vi "数据查询筛选弹框.vi"(8 "error in (no error)":errorcluster caption="错误输入（无错误）", 9 "是否初始化":enum16{"init", "keep"}(ring), 10 "database":string="database1.mdb", 11 "table":string(combo)="CODMn") -> (0 "error out":errorcluster caption="错误输出", 1 "确定输出":bool, 2 "显示项":string[](array[string]), 3 "condition":string)   [LabVIEW 2016]
uses:
  <vilib>/addons/database/Auxilliary.llb/DB Tools DataTypes.ctl
  <vilib>/picture/picture.llb/imagedata.ctl
  <vilib>/Utility/miscctls.llb/LVPointTypeDef.ctl
  <vilib>/Utility/sysdir.llb/System Directory Type.ctl
  <vilib>/addons/database/Connection.llb/DB Tools Open Connec (String).vi
  <vilib>/addons/database/Connection.llb/Conn Execute.vi
  <vilib>/addons/database/Recordset.llb/Rec Fetch Recordset Data (R).vi
  <vilib>/addons/database/Recordset.llb/Rec Destroy - Connection.vi
  <userlib>/_OpenG.lib/array/array.llb/Remove Duplicates from 1D Array (String)__ogtk.vi
  <vilib>/addons/database/_DB Variant To Data/Database Variant To Data.xnode
  <vilib>/addons/database/NI_Database_API.lvlib
panel:
  in  "背景图像":T1
  in  "实时分钟小时数据":enum32{"实时数据", "分钟数据", "小时数据"}(radio)
  in  "确定":bool
  out "自定义2single":cluster{"起始范围":string, "截止范围":string}
  out "自定义1single":cluster{"起始范围":string, "截止范围":string}
  out "自定义2筛选条件":string[](array[string])
  out "自定义1筛选条件":string[](array[string])
  in  "标签 2":string="从：\n\n\n至："
  in  "自定义数值结束 2":dbl
  in  "自定义数值起始 2":dbl
  in  "自定义结束时间 2":timestamp(xcontrol)
  in  "自定义起始时间 2":timestamp(xcontrol)
  in  "自定义 2":T2 caption="自定义"
  in  "下拉列表":string(xcontrol)
  in  "标签":string="从：\n\n\n至："
  in  "自定义数值结束":dbl
  in  "自定义数值起始":dbl
  in  "自定义结束时间":timestamp(xcontrol)
  in  "自定义起始时间":timestamp(xcontrol)
  in  "自定义":T2
  in  "下拉列表 2":string(xcontrol)
  out "type":T3[](array[typedef])
  out "所有测量模式":string[](array[string])
  out "数组":string[](array[string])
  out "columns":string[](array[string])
  in  "测量模式":T4
  in  "退出":bool
  in  "清空":bool
  in  "时间标识输入1":timestamp(xcontrol)
  in  "时间标识输入2":timestamp(xcontrol)
  # "时间"
  # "从："
  # "至："
  # "测试模式"
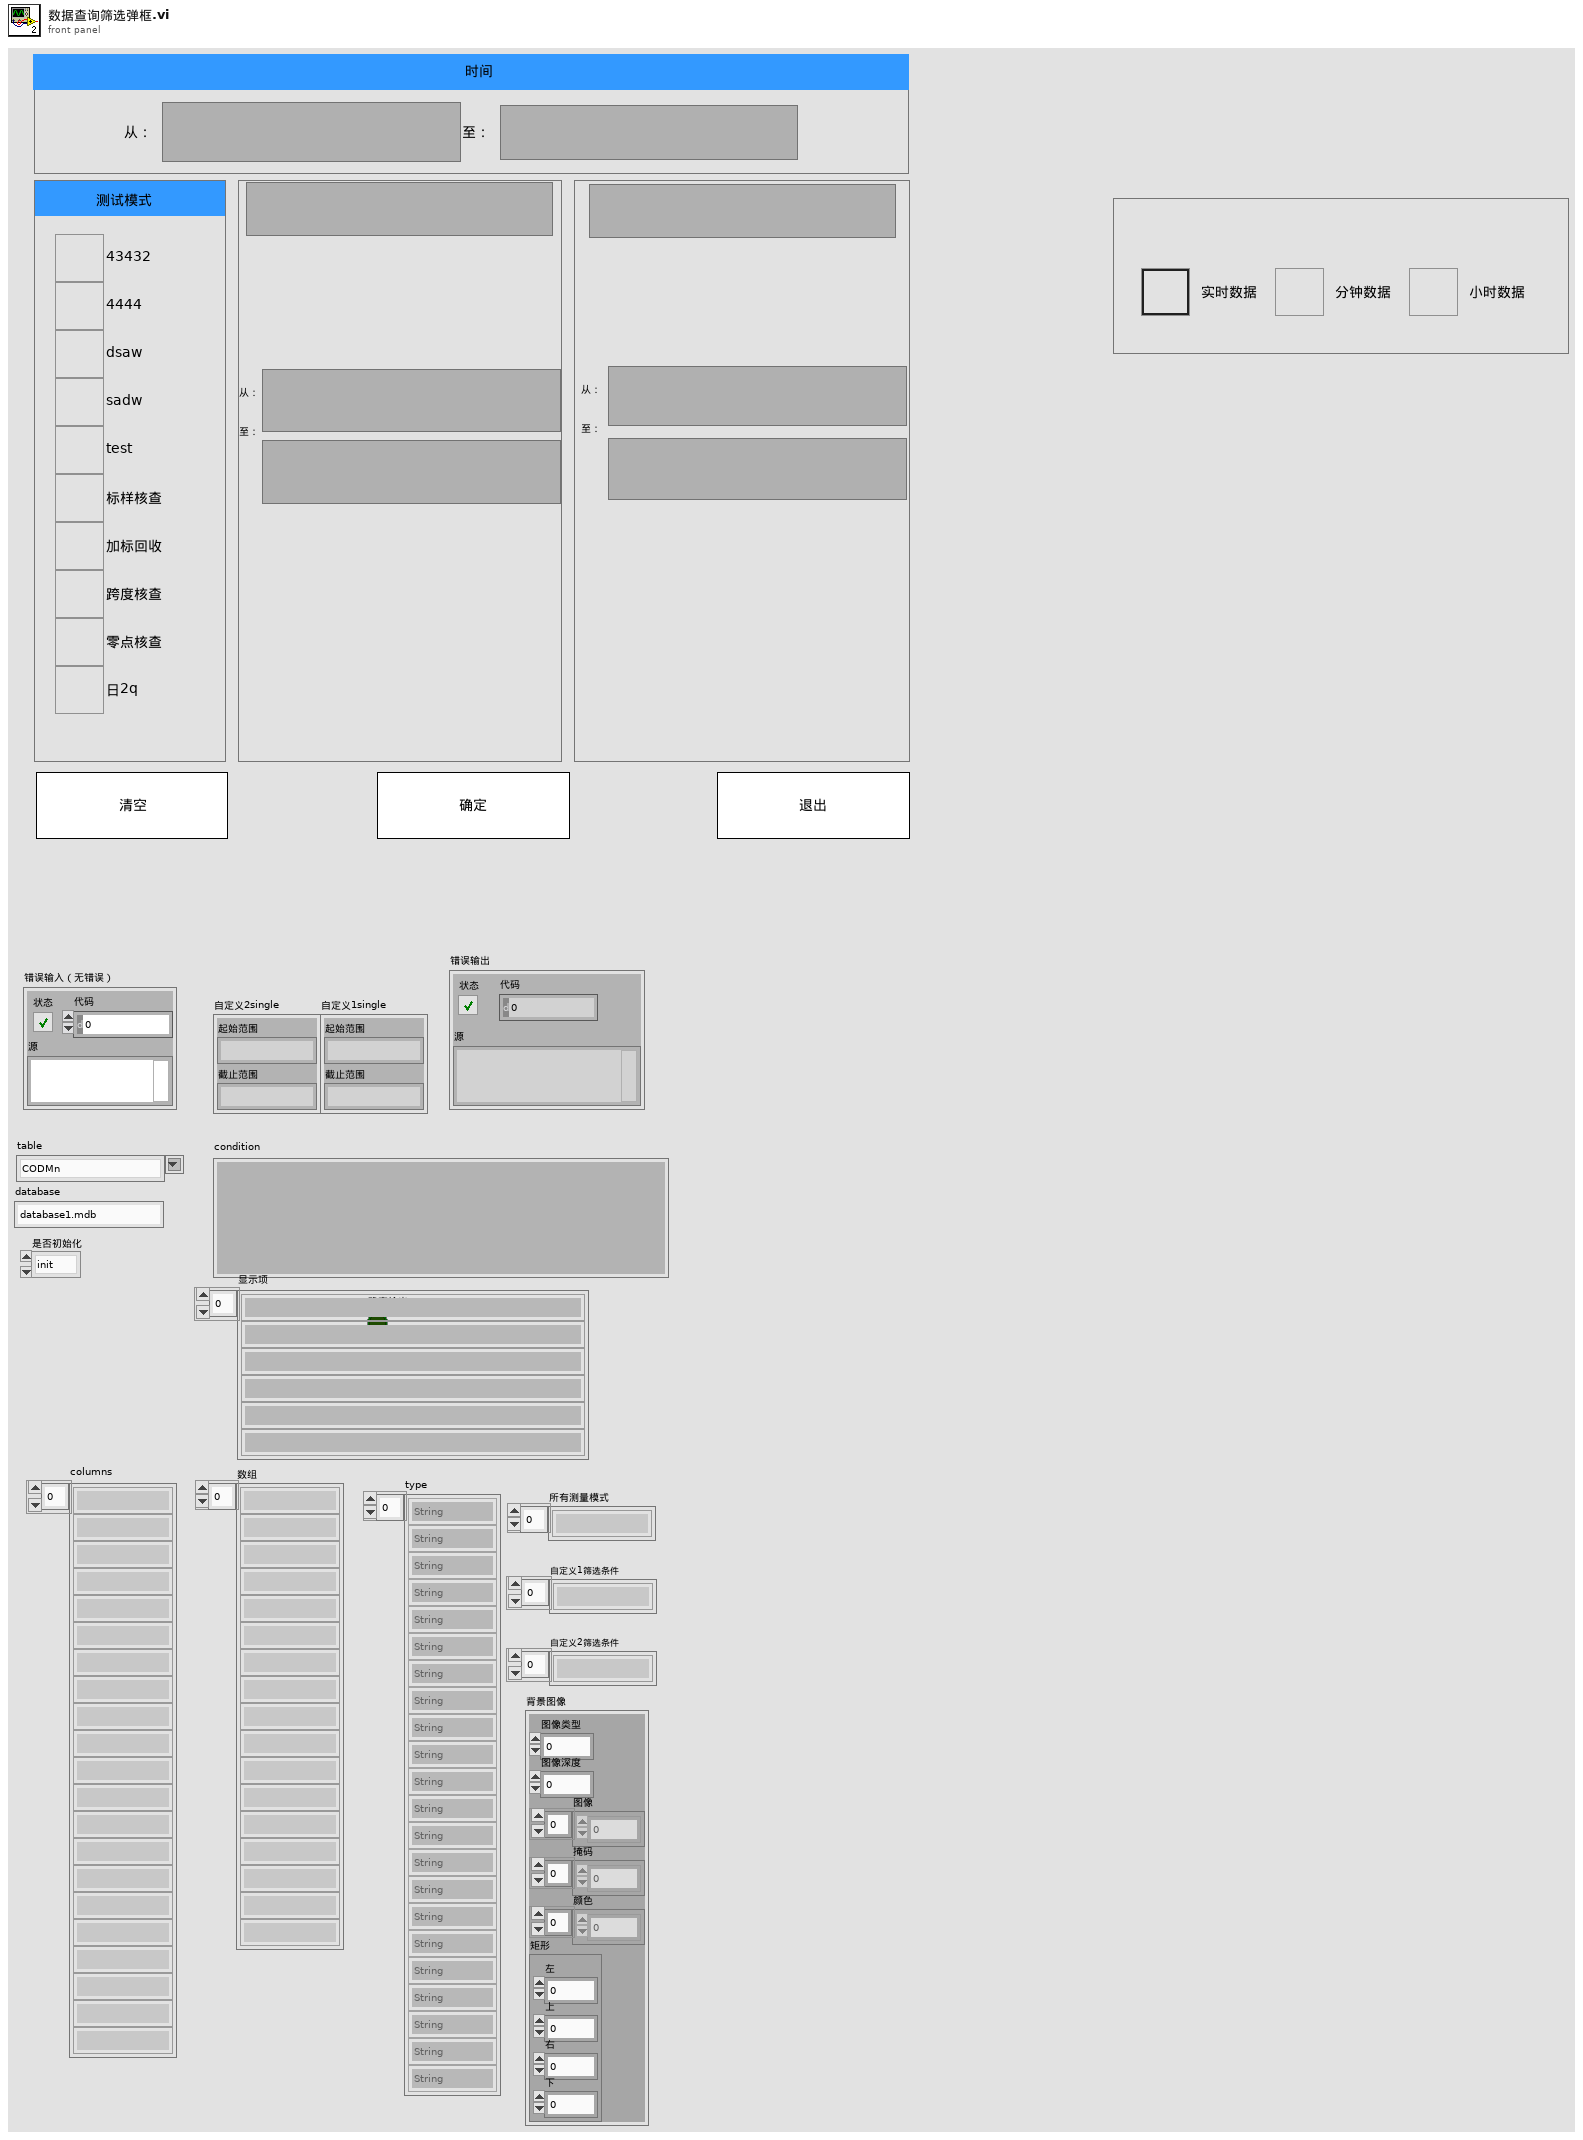
[diagram p1: front panel]
types:
  T1 = typedef "imagedata.ctl" = cluster{"image type":i32, "image depth":i32, "image":u8[], "mask":u8[], "colors":u32[], "Rectangle":cluster{"left":i16, "top":i16, "right":i16, "bottom":i16}}
  T2 = cluster{"DSADSA ":bool, "2":bool, "3":bool, "4":bool, "5":bool, "6":bool, "7":bool, "8":bool, "9":bool, "10":bool}
  T3 = typedef "NI_Database_API.lvlib/DB Tools DataTypes.ctl" = enum16{"String", "Long (I32)", "Single (SGL)", "Double (DBL)", "Date/Time", "Binary"}
  T4 = cluster{"水样测试":bool, "标样核查":bool, "零点核查":bool, "跨度核查":bool, "空白测试":bool, "平行样测试":bool, "加标回收":bool, "空白校准":bool, "标样校准":bool, "初始化清洗":bool}
  T5 = typedef "System Directory Type.ctl" = i32
  T6 = enum8{"Enabled", "Disabled", "Disabled and Grayed Out"}
  T7 = typedef "LVPointTypeDef.ctl" = cluster{"Horizontal":i16, "Vertical":i16}
  T8 = typedef "NI_Database_API.lvlib/Conn ObjectReference.ctl" = refnum<k1>
  T9 = cluster{"name":string, "database data type":T3, "defined size":i32}[]
  T10 = typedef "NI_Database_API.lvlib/Rec ObjectReference.ctl" = refnum<k1>
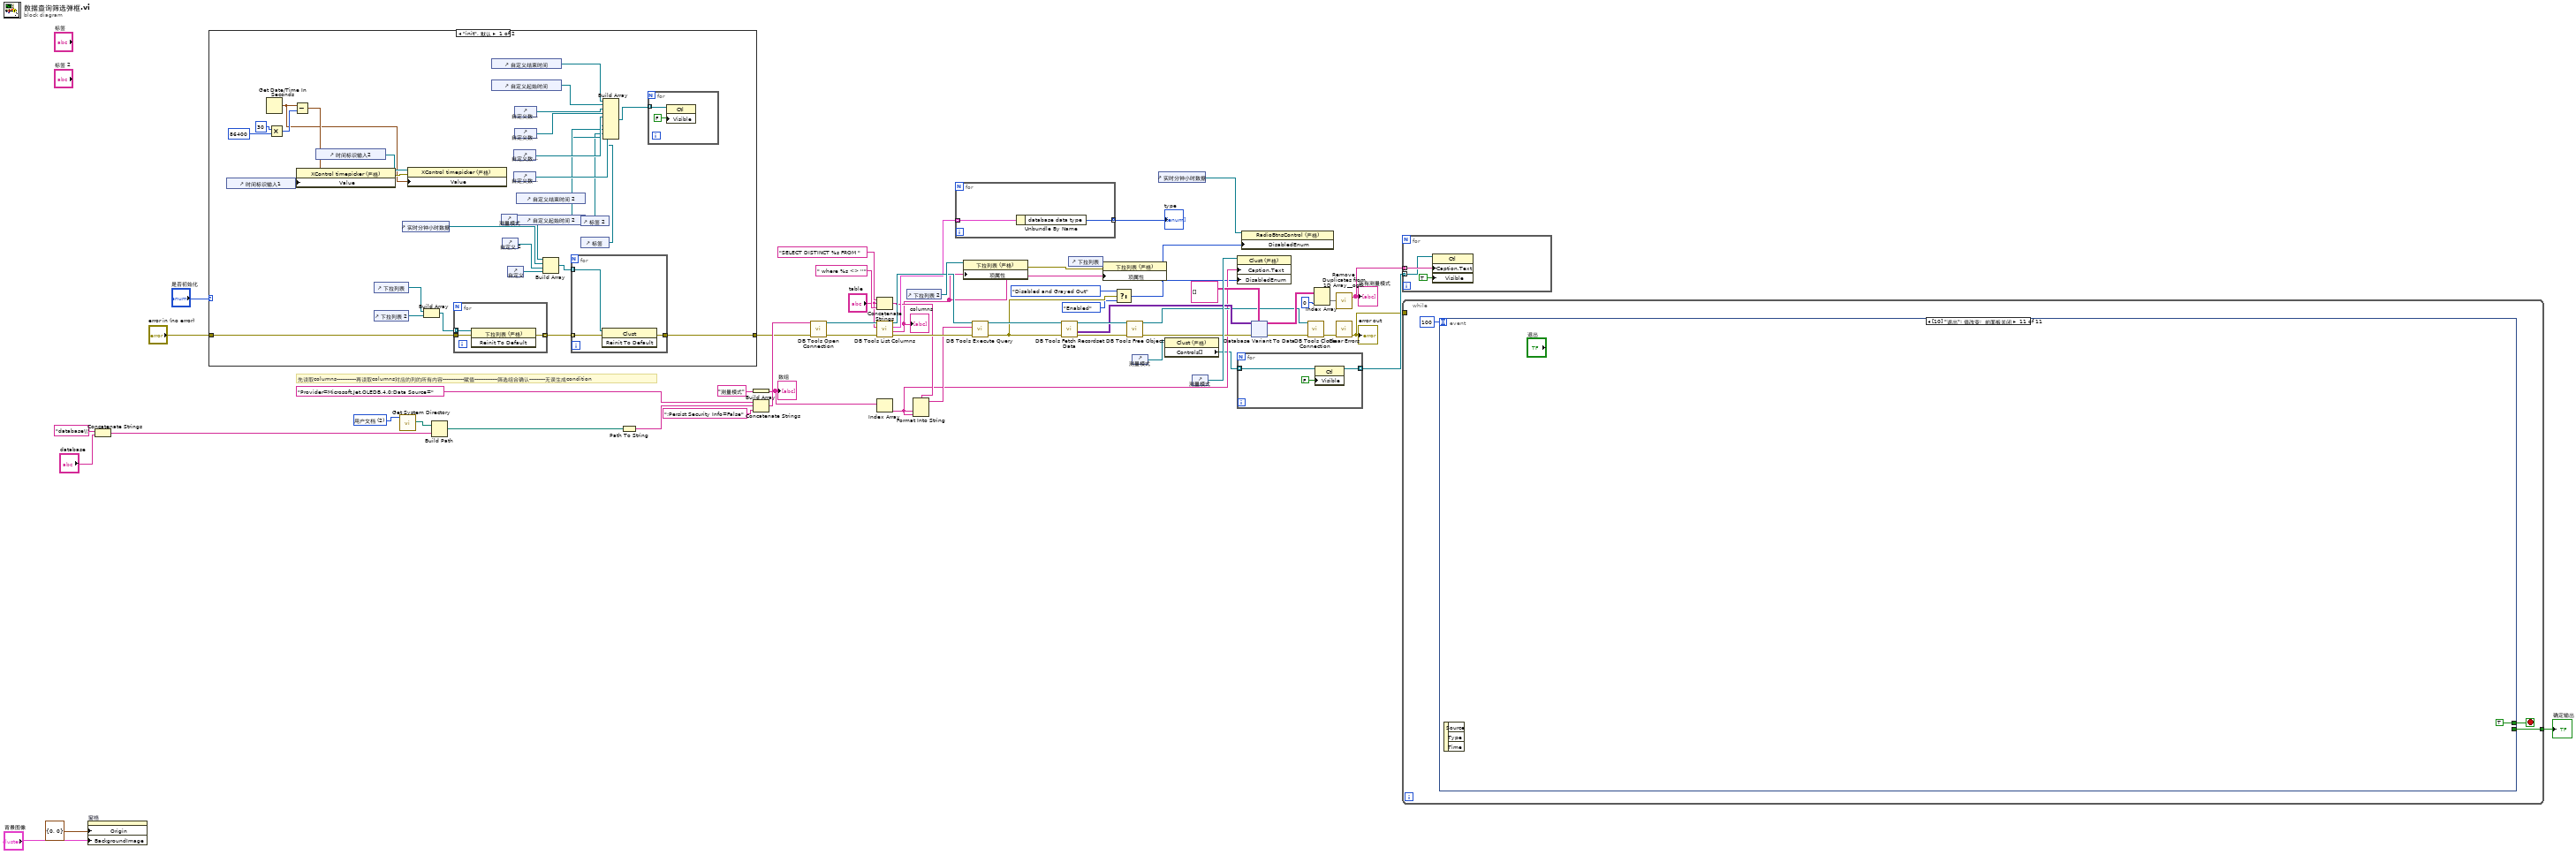
[diagram p0: block diagram]
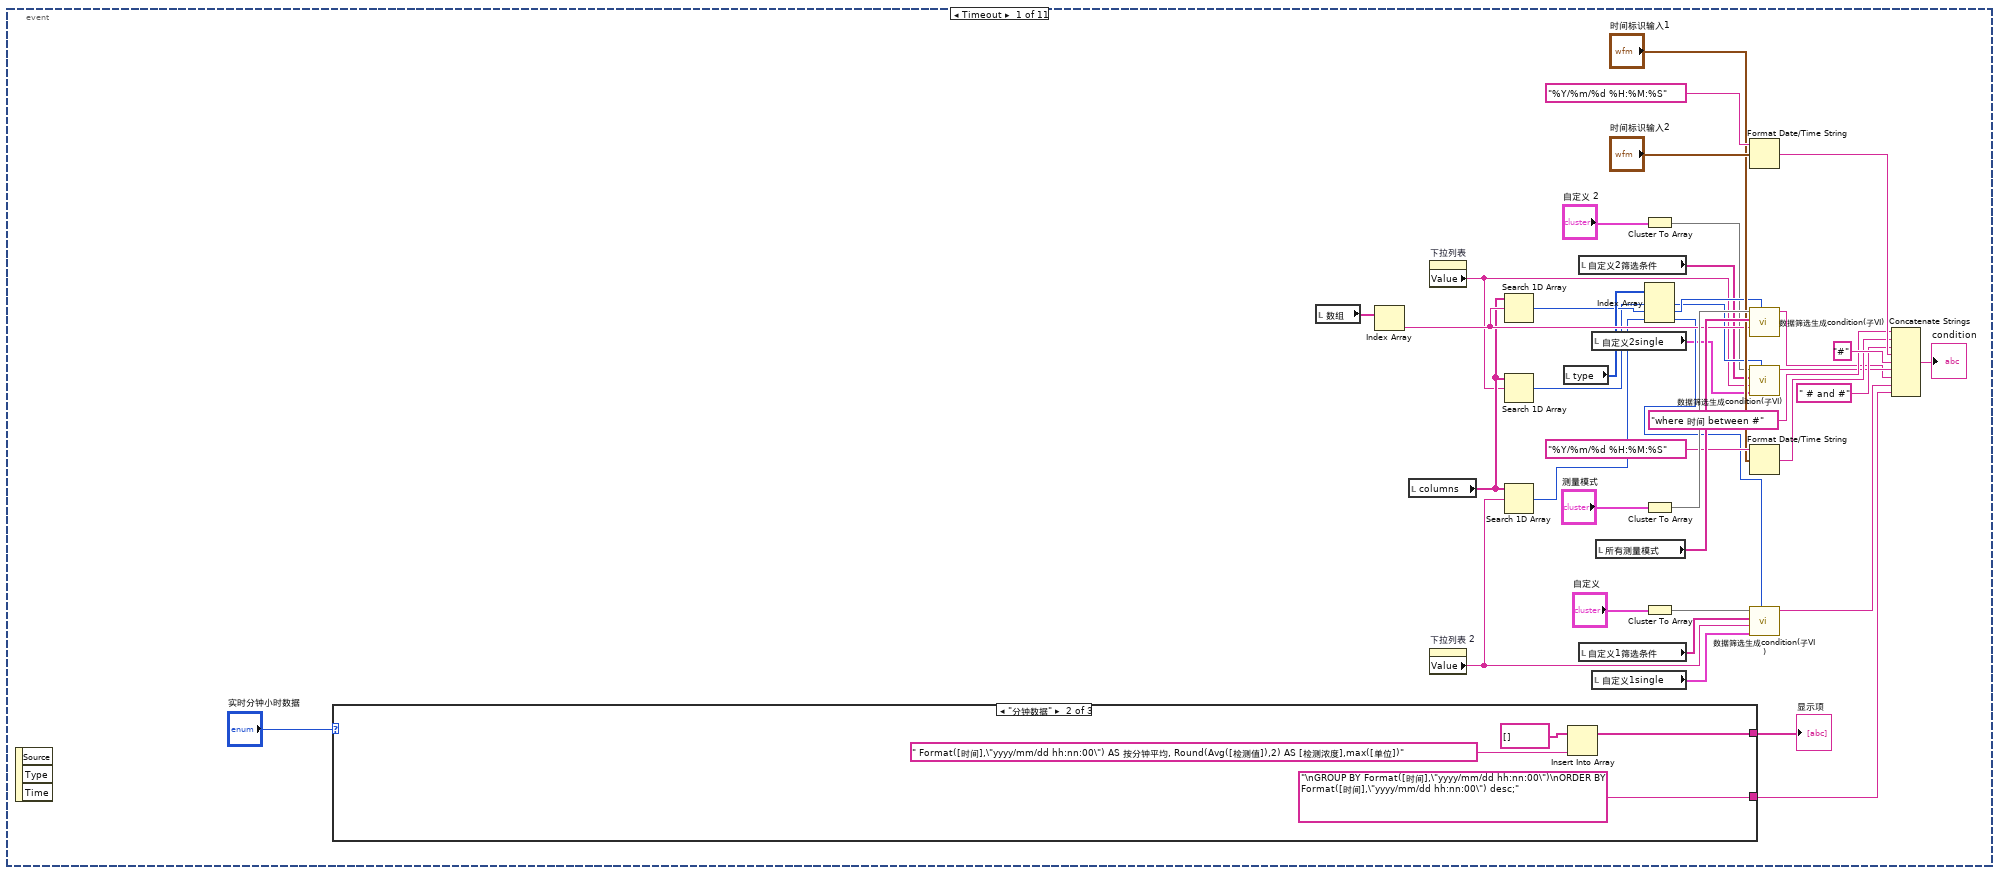
[diagram p3: hidden frame]
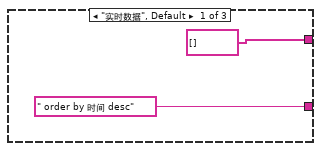
[diagram p4: hidden frame]
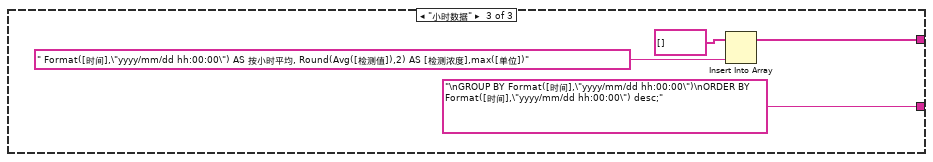
[diagram p5: hidden frame]
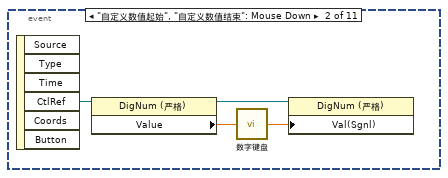
[diagram p6: hidden frame]
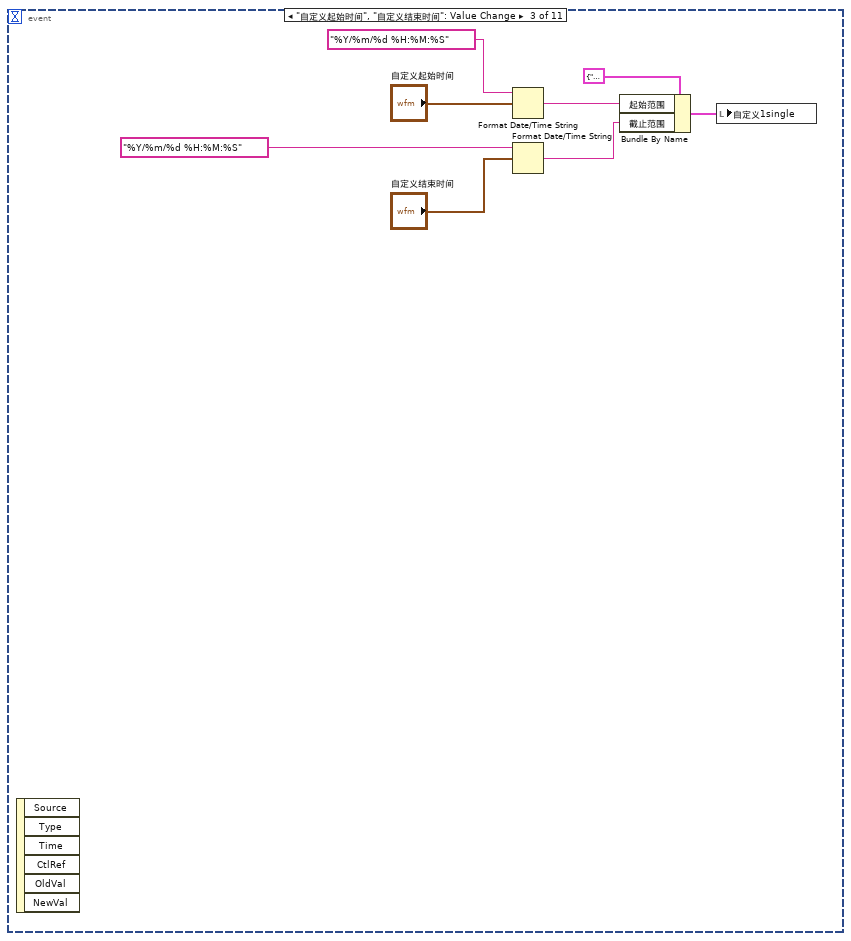
[diagram p7: hidden frame]
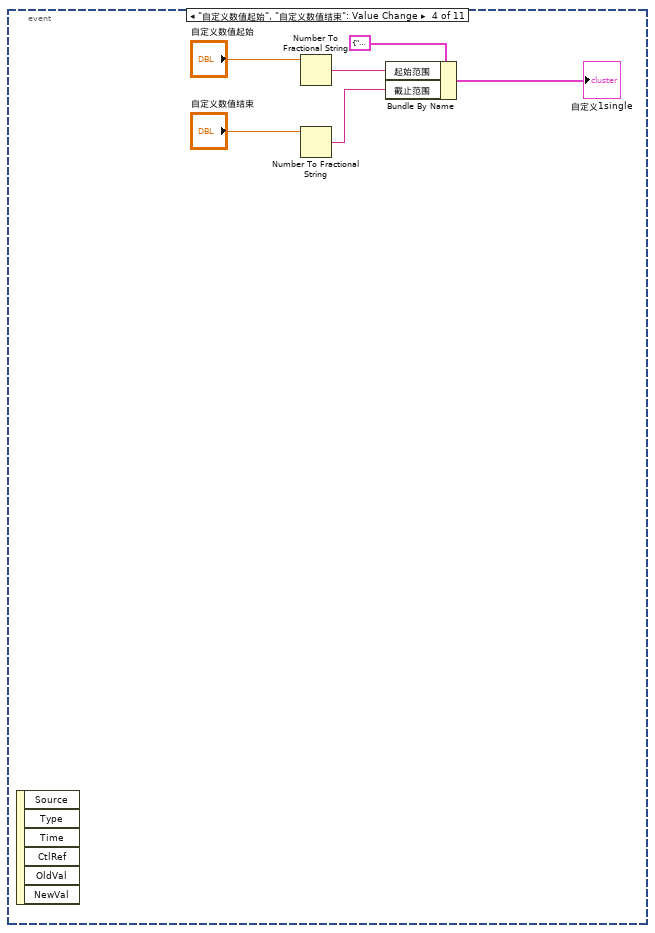
[diagram p8: hidden frame]
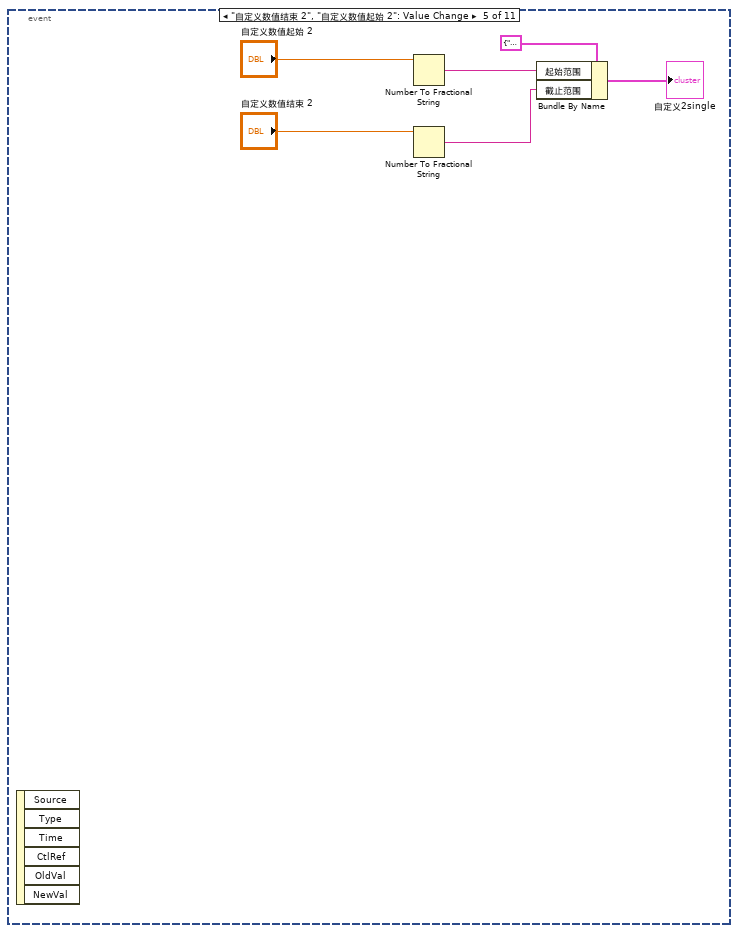
[diagram p9: hidden frame]
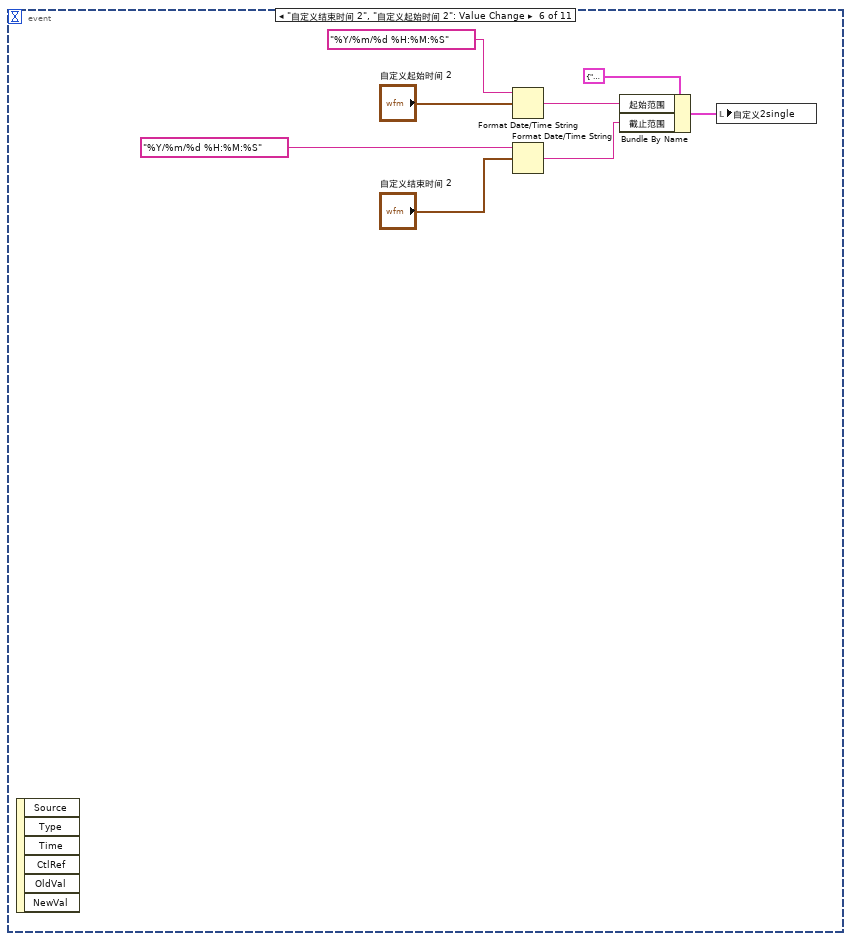
[diagram p10: hidden frame]
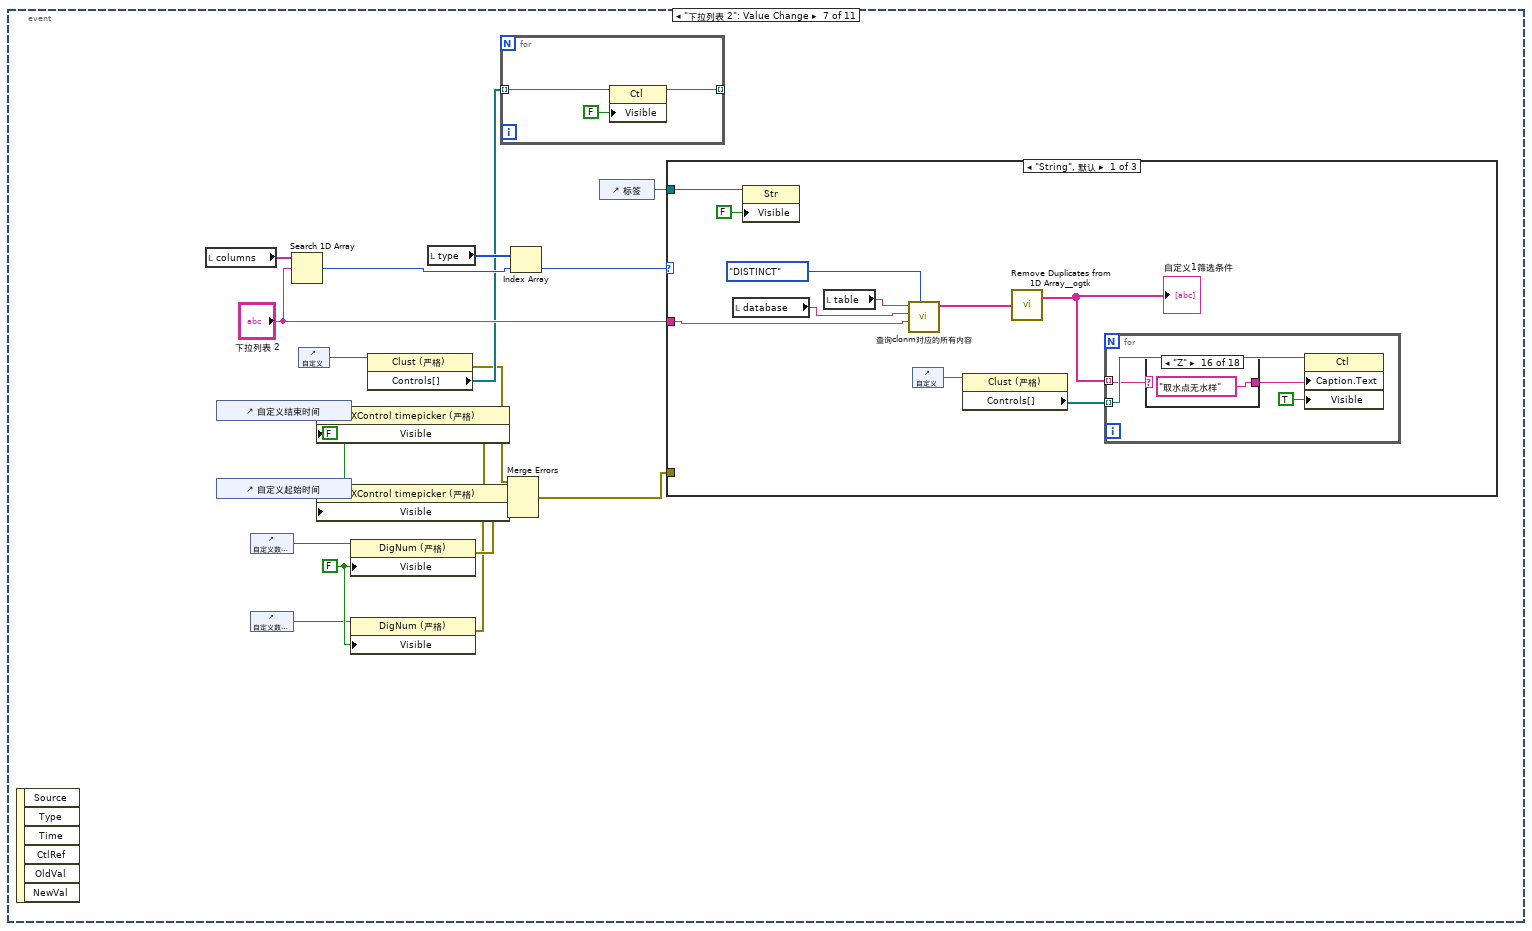
[diagram p11: hidden frame]
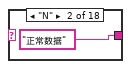
[diagram p13: hidden frame]
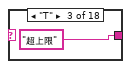
[diagram p14: hidden frame]
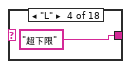
[diagram p15: hidden frame]
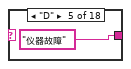
[diagram p16: hidden frame]
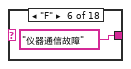
[diagram p17: hidden frame]
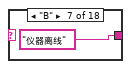
[diagram p18: hidden frame]
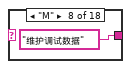
[diagram p19: hidden frame]
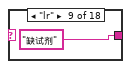
[diagram p20: hidden frame]
diagram:
  w1 = T5 2 items=["用户目录"=0, "用户桌面"=1, "用户文档"=2, "用户应用程序数据"=3, "用户设置"=4, "用户临时目录"=5, "公共文档"=6, "公共应用程序数据"=7, "公共设置"=8, "公共缓存"=13, "系统核心库"=9, "系统安装库"=10, "应用程序文件"=11, "启动盘根目录"=12] ("system directory type")
  # "先读取columns-----------再读取columns对应的列的所有内容------------赋值-------------筛选组合确认---------无误生成condition"
  n1 = property on="窗格" class="Pane"("Origin"=T7 {"Horizontal"=0, "Vertical"=0} ("原点"), "BackgroundImage"="背景图像") -> ()  [unwired: 2 in, 2 out]
  n2 = Concatenate Strings("database\\" ("名称或相对路径"), "database") -> (w50:string)
  n3 = case shown="\"init\", 默认" "是否初始化" {
    tunnel: "error in (no error)" -> [w63 w96]
    tunnel: [w82 w96] -> w10
    frame "init", Default {
      n4 = control-ref of="时间标识输入1"() -> (w65:refnum<vi>)
      n5 = Get Date/Time In Seconds() -> (seconds since 1Jan1904=w58:timestamp)
      n6 = Multiply(x=30, y=86400) -> (x*y=w77:i32)
      n7 = Subtract(x=w58, y=w77) -> (x-y=w81:timestamp)
      n8 = property class="XControl timepicker (严格)"(reference=w65, "Value"=w81) -> (error out=w80:errorcluster)  [unwired: 1 in, 1 out]
      n9 = control-ref of="时间标识输入2"() -> (w64:refnum<vi>)
      n10 = control-ref of="下拉列表"() -> (w61:refnum<vi>)
      n11 = control-ref of="下拉列表 2"() -> (w60:refnum<vi>)
      n12 = control-ref of="实时分钟小时数据"() -> (w87:refnum<vi>)
      n13 = property class="XControl timepicker (严格)"(reference=w64, error in=w80, "Value"=w58) -> ()  [unwired: 2 out]
      n14 = Build Array(w61, w60) -> (w59:refnum<vi>[])
      n15 = for {
        tunnel: w63 -> [w90]
        tunnel: [w89] -> w62 mode=indexing
        tunnel: w59 -> [w88] mode=indexing
        n16 = invoke class="下拉列表 (严格)" method="Reinit To Default"(reference=w88, error in=w90) -> (error out=w89:errorcluster)  [unwired: 1 in, 2 out]
      }
      n17 = control-ref of="自定义结束时间"() -> (w76:refnum<vi>)
      n18 = control-ref of="自定义起始时间"() -> (w75:refnum<vi>)
      n19 = control-ref of="测量模式"() -> (w83:refnum<vi>)
      n20 = control-ref of="自定义 2"() -> (w86:refnum<vi>)
      n21 = control-ref of="自定义"() -> (w85:refnum<vi>)
      n22 = control-ref of="自定义数值结束 2"() -> (w72:refnum<vi>)
      n23 = control-ref of="自定义数值起始 2"() -> (w71:refnum<vi>)
      n24 = control-ref of="自定义数值结束"() -> (w74:refnum<vi>)
      n25 = control-ref of="自定义数值起始"() -> (w73:refnum<vi>)
      n26 = control-ref of="自定义结束时间 2"() -> (w69:refnum<vi>)
      n27 = control-ref of="自定义起始时间 2"() -> (w70:refnum<vi>)
      n28 = Build Array(w83, w87, w86, w85) -> (w84:refnum<vi>[])
      n29 = for {
        tunnel: w84 -> [w95] mode=indexing
        tunnel: w62 -> [w94] mode=indexing
        tunnel: [w93] -> w82
        n30 = invoke class="Clust" method="Reinit To Default"(reference=w95, error in=w94) -> (error out=w93:errorcluster)  [unwired: 1 in, 2 out]
      }
      n31 = control-ref of="标签 2"() -> (w66:refnum<vi>)
      n32 = control-ref of="标签"() -> (w67:refnum<vi>)
      n33 = Build Array(w76, w75, w74, w73, w72, w71, w69, w70, w66, w67) -> (w68:refnum<vi>[])
      n34 = for {
        tunnel: w68 -> [w92] mode=indexing
        n35 = property class="Ctl"(reference=w92, "Visible"=FALSE ("可见")) -> ()  [unwired: 1 in, 2 out]
      }
    }
    frame "keep" {
    }
  }
  n36 = call <vilib>:"Get System Directory.vi"("system directory type"=w1) -> ("system directory"=w2:path)  [unwired: 10 in]
  n37 = Build Path(base path=w2, name or relative path=w50) -> (appended path=w49:path)
  n38 = Path To String(path=w49) -> (string=w54:string)
  n39 = Build Array("测量模式" ("Element Data")) -> (w13:string[])
  "数组" <- w13
  n40 = Concatenate Strings("Provider=Microsoft.Jet.OLEDB.4.0;Data Source=", w54, ";Persist Security Info=False") -> (w53:string)
  n41 = call-poly <vilib>:"DB Tools Open Connection.vi"("error in (no error)"=w10, "connection information"=w53) -> ("error out"=w47:errorcluster, "connection reference"=w48:T8)  [unwired: 6 in]
  n42 = Concatenate Strings("SELECT DISTINCT %s FROM " ("字符串"), "table", " where %s <> ''" ("字符串")) -> (w24:string)
  n43 = call <vilib>:"DB Tools List Columns.vi"("error in (no error)"=w47, "table"="table", "connection reference"=w48) -> ("error out"=w41:errorcluster, "columns"=w3:string[], "column information"=w28:T9, "connection reference out"=w29:T8)  [unwired: 1 in]
  "columns" <- w3
  n44 = Index Array(array=w13) -> (element=w22:string)  [unwired: 1 in]
  n45 = control-ref of="下拉列表 2"() -> (w30:refnum<vi>)
  n46 = Format Into String(format string=w24, w22, w22) -> (resulting string=w40:string)  [unwired: 2 in, 1 out]
  n47 = for {
    tunnel: w28 -> [w98] mode=indexing
    tunnel: [w97] -> w27 mode=indexing
    n48 = Unbundle By Name(w98) -> ("database data type"=w97:T3)
  }
  "type" <- w27
  n49 = property class="下拉列表 (严格)"(reference=w30, "项属性"=w3) -> (error out=w9:errorcluster)  [unwired: 1 in, 1 out]
  n50 = call-poly <vilib>:"DB Tools Execute Query.vi"("error in (no error)"=w41, "SQL query"=w40, "connection reference"=w29) -> ("error out"=w21:errorcluster, "recordset reference"=w44:T10)  [unwired: 5 in]
  n51 = call-poly <vilib>:"DB Tools Fetch Recordset Data.vi"("error in (no error)"=w21, "recordset reference"=w44) -> ("error out"=w43:errorcluster, "recordset data"=w36:variant[][], "recordset reference out"=w42:T10)  [unwired: 3 in]
  n52 = control-ref of="下拉列表"() -> (w18:refnum<vi>)
  n53 = property class="下拉列表 (严格)"(reference=w18, error in=w9, "项属性"=w3) -> ()  [unwired: 2 out]
  n54 = Select(t=T6."Disabled and Grayed Out" ("禁用"), s=w21, f=T6."Enabled" ("禁用")) -> (s? t:f=w5:T6)
  n55 = call-poly <vilib>:"DB Tools Free Object.vi"("error in (no error)"=w43, "recordset reference"=w42) -> ("error out"=w35:errorcluster, "connection reference"=w34:T8)  [unwired: 8 in]
  n56 = control-ref of="测量模式"() -> (w57:refnum<vi>)
  n57 = control-ref of="实时分钟小时数据"() -> (w6:refnum<vi>)
  n58 = property class="Clust (严格)"(reference=w57) -> ("Controls[]"=w17:refnum<vi>[])  [unwired: 1 in, 2 out]
  n59 = control-ref of="测量模式"() -> (w45:refnum<vi>)
  n60 = property class="Clust (严格)"(reference=w45, "Caption.Text"=w22, "DisabledEnum"=w5) -> ()  [unwired: 1 in, 2 out]
  n61 = for {
    tunnel: w17 -> [w101] mode=indexing
    tunnel: [w99] -> w16 mode=indexing
    n62 = property class="Ctl"(reference=w101, "Visible"=FALSE ("可见")) -> (reference out=w99:refnum<vi>)  [unwired: 1 in, 1 out]
  }
  n63 = property class="RadioBtnsControl (严格)"(reference=w6, "DisabledEnum"=w5) -> ()  [unwired: 1 in, 2 out]
  n64 = xnode "Database Variant To Data"("database variant"=w36, "error in (no error)"=w35, "type"=string[][] []) -> ("data"=w37:string[][], "error out"=w38:errorcluster)
  n65 = call <vilib>:"DB Tools Close Connection.vi"("error in (no error)"=w38, "connection reference"=w34) -> ("error out"=w12:errorcluster)  [unwired: 5 in]
  n66 = Index Array(array=w37, index (col)=0 ("禁用的索引 (列)")) -> (element=w32:string[])  [unwired: 1 in]
  n67 = call-poly <userlib>:"Remove Duplicates from 1D Array__ogtk.vi"("Input Array"=w32) -> ("Output Array"=w15:string[])  [unwired: 1 out]
  "所有测量模式" <- w15
  n68 = call <vilib>:"Clear Errors.vi"("error in (no error)"=w12) -> ("error out"=w7:errorcluster)  [unwired: 5 in, 1 out]
  "error out" <- w7
  n69 = for {
    tunnel: w15 -> [w104] mode=indexing
    tunnel: w16 -> [w102] mode=indexing
    n70 = property class="Ctl"(reference=w102, "Caption.Text"=w104, "Visible"=TRUE ("可见")) -> ()  [unwired: 1 in, 2 out]
  }
  n71 = while {
    tunnel: [w105] -> w14
    tunnel: w7 -> [_]
    stop <- w107 stop-if-true
    n72 = event shown="[10] \"退出\": 值改变;  前面板关闭" {
      selector: _ -> [_ _ _ _ _ _ _ _ _ _ _]
      dyn-events: _ -> [_ _ _ _ _ _ _ _ _ _ _]
      timeout: 100 -> [_ _ _ _ _ _ _ _ _ _ _]
      tunnel: [_ _ _ _ _ _ _ _ _ w387 TRUE] -> w107
      tunnel: [_ _ _ _ _ _ _ _ _ w387 _] -> w105
      event Timeout {
        n73 = event-data() -> ()  [unwired: 1 in, 3 out]
        n74 = case shown="\"分钟数据\"" "实时分钟小时数据" {
          tunnel: [string[] [] ("显示项") w149 w153] -> w108
          tunnel: [" order by 时间 desc" ("字符串") "\nGROUP BY Format([时间],\"yyyy/mm/dd hh:nn:00\")\nORDER BY Format([时间],\"yyyy/mm/dd hh:nn:00\") desc;" ("字符串") "\nGROUP BY Format([时间],\"yyyy/mm/dd hh:00:00\")\nORDER BY Format([时间],\"yyyy/mm/dd hh:00:00\") desc;" ("字符串")] -> w109
          frame "实时数据", Default {
          }
          frame "分钟数据" {
            n75 = Insert Into Array(array=string[] [] ("显示项"), new element=" Format([时间],\"yyyy/mm/dd hh:nn:00\") AS 按分钟平均, Round(Avg([检测值]),2) AS [检测浓度],max([单位])" ("新元素/子数组")) -> (w149:string[])  [unwired: 1 in]
          }
          frame "小时数据" {
            n76 = Insert Into Array(array=string[] [] ("显示项"), new element=" Format([时间],\"yyyy/mm/dd hh:00:00\") AS 按小时平均, Round(Avg([检测值]),2) AS [检测浓度],max([单位])" ("新元素/子数组")) -> (w153:string[])  [unwired: 1 in]
          }
        }
        "显示项" <- w108
        n77 = local read "数组"() -> (w146:string[])
        n78 = Index Array(array=w146) -> (element=w132:string)  [unwired: 1 in]
        n79 = local read "columns"() -> (w126:string[])
        n80 = property on="下拉列表" class="下拉列表 (严格)"() -> ("Value"=w117:string)  [unwired: 2 in, 2 out]
        n81 = property on="下拉列表 2" class="下拉列表 (严格)"() -> ("Value"=w116:string)  [unwired: 2 in, 2 out]
        n82 = Search 1D Array(1D array=w126, element=w132) -> (index of element=w130:i32)  [unwired: 1 in]
        n83 = Search 1D Array(1D array=w126, element=w117) -> (index of element=w125:i32)  [unwired: 1 in]
        n84 = Search 1D Array(1D array=w126, element=w116) -> (index of element=w128:i32)  [unwired: 1 in]
        n85 = local read "type"() -> (w131:T3[])
        n86 = local read "自定义2筛选条件"() -> (w114:string[])
        n87 = local read "自定义1筛选条件"() -> (w115:string[])
        n88 = local read "自定义2single"() -> (w112:cluster{"起始范围":string, "截止范围":string})
        n89 = local read "自定义1single"() -> (w111:cluster{"起始范围":string, "截止范围":string})
        n90 = local read "所有测量模式"() -> (w145:string[])
        n91 = Cluster To Array(cluster="自定义 2") -> (array=w123:bool[])
        n92 = Index Array(array=w131, index #1=w125, index #2=w130, index #3=w128) -> (element #1=w124:T3, element #2=w129:T3, element #3=w127:T3)
        n93 = Cluster To Array(cluster="测量模式") -> (array=w144:bool[])
        n94 = Cluster To Array(cluster="自定义") -> (array=w113:bool[])
        n95 = Format Date/Time String(time format string (%c)="%Y/%m/%d %H:%M:%S" ("时间格式字符串(%c)"), seconds (now)="时间标识输入2") -> (date/time string=w141:string)  [unwired: 1 in]
        n96 = call "数据筛选生成condition(子VI).vi"("database data type"=w129, "段名"=w132, "筛选内容"=w145, "簇转数组"=w144) -> ("condition"=w121:string)  [unwired: 7 in]
        n97 = call "数据筛选生成condition(子VI).vi"("database data type"=w124, "Single"=w112, "段名"=w117, "筛选内容"=w114, "簇转数组"=w123) -> ("condition"=w122:string)  [unwired: 6 in]
        n98 = Format Date/Time String(time format string (%c)="%Y/%m/%d %H:%M:%S" ("时间格式字符串(%c)"), seconds (now)="时间标识输入1") -> (date/time string=w139:string)  [unwired: 1 in]
        n99 = call "数据筛选生成condition(子VI).vi"("database data type"=w127, "Single"=w111, "段名"=w116, "筛选内容"=w115, "簇转数组"=w113) -> ("condition"=w120:string)  [unwired: 6 in]
        n100 = Concatenate Strings("where 时间 between #", w139, " # and #" ("condition"), w141, "#" ("condition"), w122, w121, w120, w109) -> (→"condition":string)
      }
      event "自定义数值起始", "自定义数值结束": Mouse Down {
        n101 = event-data() -> ("CtlRef"=w160:refnum<vi>)  [unwired: 1 in, 5 out]
        n102 = property class="DigNum (严格)"(reference=w160) -> (reference out=w158:refnum<vi>, "Value"=w159:dbl)  [unwired: 1 in, 1 out]
        n103 = call "数字键盘.vi"("OldNumber"=w159) -> ("NewNumber"=w157:sgl)
        n104 = property class="DigNum (严格)"(reference=w158, "Val(Sgnl)"=w157) -> ()  [unwired: 1 in, 2 out]
      }
      event "自定义起始时间", "自定义结束时间": Value Change {
        n105 = event-data() -> ()  [unwired: 1 in, 6 out]
        n106 = Format Date/Time String(time format string (%c)="%Y/%m/%d %H:%M:%S" ("时间格式字符串(%c)"), seconds (now)="自定义起始时间") -> (date/time string=w167:string)  [unwired: 1 in]
        n107 = Format Date/Time String(time format string (%c)="%Y/%m/%d %H:%M:%S" ("时间格式字符串(%c)"), seconds (now)="自定义结束时间") -> (date/time string=w168:string)  [unwired: 1 in]
        n108 = Bundle By Name(cluster=cluster{"起始范围":string, "截止范围":string} {"起始范围"="2", "截止范围"="5"} ("Single"), "起始范围"=w167, "截止范围"=w168) -> (w161:cluster{"起始范围":string, "截止范围":string})
        n109 = local write "自定义1single"(w161) -> ()
      }
      event "自定义数值起始", "自定义数值结束": Value Change {
        n110 = event-data() -> ()  [unwired: 1 in, 6 out]
        n111 = Number To Fractional String(number="自定义数值起始") -> (F-format string=w173:string)  [unwired: 3 in]
        n112 = Number To Fractional String(number="自定义数值结束") -> (F-format string=w174:string)  [unwired: 3 in]
        n113 = Bundle By Name(cluster=cluster{"起始范围":string, "截止范围":string} {"起始范围"="2", "截止范围"="5"} ("Single"), "起始范围"=w173, "截止范围"=w174) -> (→"自定义1single":cluster{"起始范围":string, "截止范围":string})
      }
      event "自定义数值结束 2", "自定义数值起始 2": Value Change {
        n114 = event-data() -> ()  [unwired: 1 in, 6 out]
        n115 = Number To Fractional String(number="自定义数值起始 2") -> (F-format string=w177:string)  [unwired: 3 in]
        n116 = Number To Fractional String(number="自定义数值结束 2") -> (F-format string=w176:string)  [unwired: 3 in]
        n117 = Bundle By Name(cluster=cluster{"起始范围":string, "截止范围":string} {"起始范围"="2", "截止范围"="5"} ("Single"), "起始范围"=w177, "截止范围"=w176) -> (→"自定义2single":cluster{"起始范围":string, "截止范围":string})
      }
      event "自定义结束时间 2", "自定义起始时间 2": Value Change {
        n118 = event-data() -> ()  [unwired: 1 in, 6 out]
        n119 = Format Date/Time String(time format string (%c)="%Y/%m/%d %H:%M:%S" ("时间格式字符串(%c)"), seconds (now)="自定义起始时间 2") -> (date/time string=w186:string)  [unwired: 1 in]
        n120 = Format Date/Time String(time format string (%c)="%Y/%m/%d %H:%M:%S" ("时间格式字符串(%c)"), seconds (now)="自定义结束时间 2") -> (date/time string=w187:string)  [unwired: 1 in]
        n121 = Bundle By Name(cluster=cluster{"起始范围":string, "截止范围":string} {"起始范围"="2", "截止范围"="5"} ("Single"), "起始范围"=w186, "截止范围"=w187) -> (w188:cluster{"起始范围":string, "截止范围":string})
        n122 = local write "自定义2single"(w188) -> ()
      }
      event "下拉列表 2": Value Change {
        w199 = FALSE ("可见")
        w189 = FALSE ("可见")
        n123 = event-data() -> ()  [unwired: 1 in, 6 out]
        n124 = local read "columns"() -> (w206:string[])
        n125 = control-ref of="自定义结束时间"() -> (w201:refnum<vi>)
        n126 = control-ref of="自定义起始时间"() -> (w200:refnum<vi>)
        n127 = control-ref of="自定义数值结束"() -> (w198:refnum<vi>)
        n128 = control-ref of="自定义数值起始"() -> (w191:refnum<vi>)
        n129 = Search 1D Array(1D array=w206, element="下拉列表 2") -> (index of element=w208:i32)  [unwired: 1 in]
        n130 = control-ref of="自定义"() -> (w203:refnum<vi>)
        n131 = property class="XControl timepicker (严格)"(reference=w201, "Visible"=w189) -> (error out=w196:errorcluster)  [unwired: 1 in, 1 out]
        n132 = property class="XControl timepicker (严格)"(reference=w200, "Visible"=w189) -> (error out=w195:errorcluster)  [unwired: 1 in, 1 out]
        n133 = property class="DigNum (严格)"(reference=w198, "Visible"=w199) -> (error out=w194:errorcluster)  [unwired: 1 in, 1 out]
        n134 = property class="DigNum (严格)"(reference=w191, "Visible"=w199) -> (error out=w193:errorcluster)  [unwired: 1 in, 1 out]
        n135 = property class="Clust (严格)"(reference=w203) -> (error out=w197:errorcluster, "Controls[]"=w202:refnum<vi>[])  [unwired: 1 in, 1 out]
        n136 = local read "type"() -> (w207:T3[])
        n137 = for {
          tunnel: w202 -> [w211] mode=indexing
          tunnel: [w209] -> _ mode=indexing
          n138 = property class="Ctl"(reference=w211, "Visible"=FALSE ("可见")) -> (reference out=w209:refnum<vi>)  [unwired: 1 in, 1 out]
        }
        n139 = Merge Errors(w197, w196, w195, w194, w193) -> (w192:errorcluster)
        n140 = Index Array(array=w207, index=w208) -> (element=w204:T3)
        n141 = control-ref of="标签"() -> (w190:refnum<vi>)
        n142 = case shown="\"String\", 默认" w204 {
          tunnel: "下拉列表 2" -> [w219 w251 w272]
          tunnel: w192 -> [_ _ _]
          tunnel: w190 -> [w214 w257 w277]
          frame "String", Default {
            n143 = local read "database"() -> (w220:string)
            n144 = property class="Str"(reference=w214, "Visible"=FALSE ("可见")) -> ()  [unwired: 1 in, 2 out]
            n145 = local read "table"() -> (w221:string)
            n146 = call "查询clonm对应的所有内容.vi"("条件"=enum16{"DISTINCT", "MIN", "MAX"}."DISTINCT", "组合框"=w219, "database"=w220, "table"=w221) -> ("输出数组"=w218:string[])  [unwired: 6 in, 1 out]
            n147 = control-ref of="自定义"() -> (w216:refnum<vi>)
            n148 = property class="Clust (严格)"(reference=w216) -> ("Controls[]"=w215:refnum<vi>[])  [unwired: 1 in, 2 out]
            n149 = call-poly <userlib>:"Remove Duplicates from 1D Array__ogtk.vi"("Input Array"=w218) -> ("Output Array"=w217:string[])  [unwired: 1 out]
            "自定义1筛选条件" <- w217
            n150 = for {
              tunnel: w217 -> [w222] mode=indexing
              tunnel: w215 -> [w224] mode=indexing
              n151 = case shown="\"Z\"" w222 {
                selector: w222 -> [w226 _ _ _ _ _ _ _ _ _ _ _ _ _ _ _ _ _]
                tunnel: [w226 "正常数据" "超上限" "超下限" "仪器故障" "仪器通信故障" "仪器离线" "维护调试数据" "缺试剂" "缺纯水" "缺水样" "缺标液" "加标回收" "平行样测试" "电源故障" "取水点无水样" "手工输入数据" "手动测试数据"] -> w223
                frame Default {
                }
                frame "N" {
                }
                frame "T" {
                }
                frame "L" {
                }
                frame "D" {
                }
                frame "F" {
                }
                frame "B" {
                }
                frame "M" {
                }
                frame "lr" {
                }
                frame "lp" {
                }
                frame "lw" {
                }
                frame "ls" {
                }
                frame "ra" {
                }
                frame "pt" {
                }
                frame "P" {
                }
                frame "Z" {
                }
                frame "S" {
                }
                frame "hd" {
                }
              }
              n152 = property class="Ctl"(reference=w224, "Caption.Text"=w223, "Visible"=TRUE ("可见")) -> ()  [unwired: 1 in, 2 out]
            }
          }
          frame "Long (I32)".."Double (DBL)" {
            w259 = TRUE ("可见")
            n153 = local read "database"() -> (w252:string)
            n154 = property class="Str"(reference=w257, "Visible"=TRUE ("可见")) -> ()  [unwired: 1 in, 2 out]
            n155 = local read "table"() -> (w253:string)
            n156 = call "查询clonm对应的所有内容.vi"("条件"=enum16{"DISTINCT", "MIN", "MAX"}."MAX", "组合框"=w251, "database"=w252, "table"=w253) -> ("输出数组"=w250:string[])  [unwired: 6 in, 1 out]
            n157 = call "查询clonm对应的所有内容.vi"("条件"=enum16{"DISTINCT", "MIN", "MAX"}."MIN", "组合框"=w251, "database"=w252, "table"=w253) -> ("输出数组"=w255:string[])  [unwired: 6 in, 1 out]
            n158 = Index Array(array=w250) -> (element=w245:string)  [unwired: 1 in]
            n159 = Index Array(array=w255) -> (element=w244:string)  [unwired: 1 in]
            n160 = control-ref of="自定义数值结束"() -> (w260:refnum<vi>)
            n161 = control-ref of="自定义数值起始"() -> (w261:refnum<vi>)
            n162 = Fract/Exp String To Number(string=w245) -> (number=w248:dbl)  [unwired: 3 in, 1 out]
            n163 = Fract/Exp String To Number(string=w244) -> (number=w249:dbl)  [unwired: 3 in, 1 out]
            n164 = Bundle By Name(cluster=cluster{"起始范围":string, "截止范围":string} {"起始范围"="2", "截止范围"="5"} ("Single"), "起始范围"=w244, "截止范围"=w245) -> (w246:cluster{"起始范围":string, "截止范围":string})
            n165 = property class="DigNum (严格)"(reference=w260, "Visible"=w259, "Value"=w248) -> ()  [unwired: 1 in, 2 out]
            n166 = property class="DigNum (严格)"(reference=w261, "Visible"=w259, "Value"=w249) -> ()  [unwired: 1 in, 2 out]
            n167 = local write "自定义1single"(w246) -> ()
          }
          frame "Date/Time" {
            n168 = local read "database"() -> (w273:string)
            n169 = property class="Str"(reference=w277, "Visible"=TRUE ("可见")) -> ()  [unwired: 1 in, 2 out]
            n170 = local read "table"() -> (w274:string)
            n171 = call "查询clonm对应的所有内容.vi"("条件"=enum16{"DISTINCT", "MIN", "MAX"}."MAX", "组合框"=w272, "database"=w273, "table"=w274) -> ("输出数组"=w271:string[])  [unwired: 6 in, 1 out]
            n172 = call "查询clonm对应的所有内容.vi"("条件"=enum16{"DISTINCT", "MIN", "MAX"}."MIN", "组合框"=w272, "database"=w273, "table"=w274) -> ("输出数组"=w266:string[])  [unwired: 6 in, 1 out]
            n173 = Index Array(array=w271) -> (element=w265:string)  [unwired: 1 in]
            n174 = Index Array(array=w266) -> (element=w263:string)  [unwired: 1 in]
            n175 = call "格式日期时间字符串.vi"("data[0]"=w265) -> ("日期/时间字符串"=w264:string)  [unwired: 10 in]
            n176 = call "格式日期时间字符串.vi"("data[0]"=w263) -> ("日期/时间字符串"=w262:string)  [unwired: 10 in]
            n177 = control-ref of="自定义起始时间"() -> (w279:refnum<vi>)
            n178 = control-ref of="自定义结束时间"() -> (w280:refnum<vi>)
            n179 = call "日期字符串格式至时间格式转换(子VI).vi"("data[0]"=w264) -> ("time stamp"=w269:timestamp)  [unwired: 10 in]
            n180 = call "日期字符串格式至时间格式转换(子VI).vi"("data[0]"=w262) -> ("time stamp"=w270:timestamp)  [unwired: 10 in]
            n181 = Bundle By Name(cluster=cluster{"起始范围":string, "截止范围":string} {"起始范围"="2", "截止范围"="5"} ("Single"), "起始范围"=w262, "截止范围"=w264) -> (w267:cluster{"起始范围":string, "截止范围":string})
            n182 = property class="XControl timepicker (严格)"(reference=w279, "Visible"=TRUE ("可见"), "Value"=w270) -> ()  [unwired: 1 in, 2 out]
            n183 = property class="XControl timepicker (严格)"(reference=w280, "Visible"=TRUE ("可见"), "Value"=w269) -> ()  [unwired: 1 in, 2 out]
            n184 = local write "自定义1single"(w267) -> ()
          }
        }
      }
      event "下拉列表": Value Change {
        w293 = FALSE ("可见")
        w283 = FALSE ("可见")
        n185 = event-data() -> ()  [unwired: 1 in, 6 out]
        n186 = local read "columns"() -> (w299:string[])
        n187 = control-ref of="自定义结束时间 2"() -> (w295:refnum<vi>)
        n188 = control-ref of="自定义起始时间 2"() -> (w294:refnum<vi>)
        n189 = control-ref of="自定义数值结束 2"() -> (w292:refnum<vi>)
        n190 = control-ref of="自定义数值起始 2"() -> (w285:refnum<vi>)
        n191 = control-ref of="自定义 2"() -> (w297:refnum<vi>)
        n192 = Search 1D Array(1D array=w299, element="下拉列表") -> (index of element=w301:i32)  [unwired: 1 in]
        n193 = property class="XControl timepicker (严格)"(reference=w295, "Visible"=w283) -> (error out=w290:errorcluster)  [unwired: 1 in, 1 out]
        n194 = property class="XControl timepicker (严格)"(reference=w294, "Visible"=w283) -> (error out=w289:errorcluster)  [unwired: 1 in, 1 out]
        n195 = property class="DigNum (严格)"(reference=w292, "Visible"=w293) -> (error out=w288:errorcluster)  [unwired: 1 in, 1 out]
        n196 = property class="DigNum (严格)"(reference=w285, "Visible"=w293) -> (error out=w287:errorcluster)  [unwired: 1 in, 1 out]
        n197 = property class="Clust (严格)"(reference=w297) -> (error out=w291:errorcluster, "Controls[]"=w296:refnum<vi>[])  [unwired: 1 in, 1 out]
        n198 = local read "type"() -> (w300:T3[])
        n199 = for {
          tunnel: w296 -> [w305] mode=indexing
          tunnel: [w303] -> _ mode=indexing
          n200 = property class="Ctl"(reference=w305, "Visible"=FALSE ("可见")) -> (reference out=w303:refnum<vi>)  [unwired: 1 in, 1 out]
        }
        n201 = Merge Errors(w291, w290, w289, w288, w287) -> (w286:errorcluster)
        n202 = Index Array(array=w300, index=w301) -> (element=w298:T3)
        n203 = control-ref of="标签 2"() -> (w284:refnum<vi>)
        n204 = case shown="\"Long (I32)\"..\"Double (DBL)\"" w298 {
          tunnel: "下拉列表" -> [w313 w346 w364]
          tunnel: w286 -> [_ _ _]
          tunnel: w284 -> [w309 w351 w371]
          frame "String", Default {
            n205 = local read "database"() -> (w314:string)
            n206 = property class="Str"(reference=w309, "Visible"=FALSE ("可见")) -> ()  [unwired: 1 in, 2 out]
            n207 = local read "table"() -> (w315:string)
            n208 = control-ref of="自定义 2"() -> (w311:refnum<vi>)
            n209 = call "查询clonm对应的所有内容.vi"("条件"=enum16{"DISTINCT", "MIN", "MAX"}."DISTINCT", "组合框"=w313, "database"=w314, "table"=w315) -> ("输出数组"=w312:string[])  [unwired: 6 in, 1 out]
            n210 = property class="Clust (严格)"(reference=w311) -> ("Controls[]"=w310:refnum<vi>[])  [unwired: 1 in, 2 out]
            n211 = call-poly <userlib>:"Remove Duplicates from 1D Array__ogtk.vi"("Input Array"=w312) -> ("Output Array"=w306:string[])  [unwired: 1 out]
            "自定义2筛选条件" <- w306
            n212 = for {
              tunnel: w306 -> [w317] mode=indexing
              tunnel: w310 -> [w318] mode=indexing
              n213 = case shown="\"Z\"" w317 {
                selector: w317 -> [w320 _ _ _ _ _ _ _ _ _ _ _ _ _ _ _ _ _]
                tunnel: [w320 "正常数据" "超上限" "超下限" "仪器故障" "仪器通信故障" "仪器离线" "维护调试数据" "缺试剂" "缺纯水" "缺水样" "缺标液" "加标回收" "平行样测试" "电源故障" "取水点无水样" "手工输入数据" "手动测试数据"] -> w316
                frame Default {
                }
                frame "N" {
                }
                frame "T" {
                }
                frame "L" {
                }
                frame "D" {
                }
                frame "F" {
                }
                frame "B" {
                }
                frame "M" {
                }
                frame "lr" {
                }
                frame "lp" {
                }
                frame "lw" {
                }
                frame "ls" {
                }
                frame "ra" {
                }
                frame "pt" {
                }
                frame "P" {
                }
                frame "Z" {
                }
                frame "S" {
                }
                frame "hd" {
                }
              }
              n214 = property class="Ctl"(reference=w318, "Caption.Text"=w316, "Visible"=TRUE ("可见")) -> ()  [unwired: 1 in, 2 out]
            }
          }
          frame "Long (I32)".."Double (DBL)" {
            w353 = TRUE ("可见")
            n215 = local read "database"() -> (w347:string)
            n216 = property class="Str"(reference=w351, "Visible"=TRUE ("可见")) -> ()  [unwired: 1 in, 2 out]
            n217 = local read "table"() -> (w348:string)
            n218 = call "查询clonm对应的所有内容.vi"("条件"=enum16{"DISTINCT", "MIN", "MAX"}."MAX", "组合框"=w346, "database"=w347, "table"=w348) -> ("输出数组"=w345:string[])  [unwired: 6 in, 1 out]
            n219 = call "查询clonm对应的所有内容.vi"("条件"=enum16{"DISTINCT", "MIN", "MAX"}."MIN", "组合框"=w346, "database"=w347, "table"=w348) -> ("输出数组"=w340:string[])  [unwired: 6 in, 1 out]
            n220 = Index Array(array=w345) -> (element=w338:string)  [unwired: 1 in]
            n221 = Index Array(array=w340) -> (element=w339:string)  [unwired: 1 in]
            n222 = control-ref of="自定义数值结束 2"() -> (w354:refnum<vi>)
            n223 = control-ref of="自定义数值起始 2"() -> (w355:refnum<vi>)
            n224 = Fract/Exp String To Number(string=w338) -> (number=w343:dbl)  [unwired: 3 in, 1 out]
            n225 = Fract/Exp String To Number(string=w339) -> (number=w344:dbl)  [unwired: 3 in, 1 out]
            n226 = Bundle By Name(cluster=cluster{"起始范围":string, "截止范围":string} {"起始范围"="2", "截止范围"="5"} ("Single"), "起始范围"=w339, "截止范围"=w338) -> (w342:cluster{"起始范围":string, "截止范围":string})
            n227 = property class="DigNum (严格)"(reference=w354, "Visible"=w353, "Value"=w343) -> ()  [unwired: 1 in, 2 out]
            n228 = property class="DigNum (严格)"(reference=w355, "Visible"=w353, "Value"=w344) -> ()  [unwired: 1 in, 2 out]
            n229 = local write "自定义2single"(w342) -> ()
          }
          frame "Date/Time" {
            n230 = local read "database"() -> (w367:string)
            n231 = property class="Str"(reference=w371, "Visible"=TRUE ("可见")) -> ()  [unwired: 1 in, 2 out]
            n232 = local read "table"() -> (w368:string)
            n233 = call "查询clonm对应的所有内容.vi"("条件"=enum16{"DISTINCT", "MIN", "MAX"}."MAX", "组合框"=w364, "database"=w367, "table"=w368) -> ("输出数组"=w366:string[])  [unwired: 6 in, 1 out]
            n234 = call "查询clonm对应的所有内容.vi"("条件"=enum16{"DISTINCT", "MIN", "MAX"}."MIN", "组合框"=w364, "database"=w367, "table"=w368) -> ("输出数组"=w365:string[])  [unwired: 6 in, 1 out]
            n235 = Index Array(array=w366) -> (element=w359:string)  [unwired: 1 in]
            n236 = Index Array(array=w365) -> (element=w357:string)  [unwired: 1 in]
            n237 = call "格式日期时间字符串.vi"("data[0]"=w359) -> ("日期/时间字符串"=w358:string)  [unwired: 10 in]
            n238 = call "格式日期时间字符串.vi"("data[0]"=w357) -> ("日期/时间字符串"=w356:string)  [unwired: 10 in]
            n239 = control-ref of="自定义起始时间 2"() -> (w373:refnum<vi>)
            n240 = control-ref of="自定义结束时间 2"() -> (w374:refnum<vi>)
            n241 = call "日期字符串格式至时间格式转换(子VI).vi"("data[0]"=w358) -> ("time stamp"=w363:timestamp)  [unwired: 10 in]
            n242 = call "日期字符串格式至时间格式转换(子VI).vi"("data[0]"=w356) -> ("time stamp"=w362:timestamp)  [unwired: 10 in]
            n243 = Bundle By Name(cluster=cluster{"起始范围":string, "截止范围":string} {"起始范围"="2", "截止范围"="5"} ("Single"), "起始范围"=w356, "截止范围"=w358) -> (w361:cluster{"起始范围":string, "截止范围":string})
            n244 = property class="XControl timepicker (严格)"(reference=w374, "Visible"=TRUE ("可见"), "Value"=w363) -> ()  [unwired: 1 in, 2 out]
            n245 = property class="XControl timepicker (严格)"(reference=w373, "Visible"=TRUE ("可见"), "Value"=w362) -> ()  [unwired: 1 in, 2 out]
            n246 = local write "自定义2single"(w361) -> ()
          }
        }
      }
      event "清空": Value Change {
        n247 = event-data() -> ()  [unwired: 1 in, 6 out]
        n248 = control-ref of="实时分钟小时数据"() -> (w380:refnum<vi>)
        n249 = control-ref of="下拉列表"() -> (w379:refnum<vi>)
        n250 = control-ref of="下拉列表 2"() -> (w378:refnum<vi>)
        n251 = control-ref of="测量模式"() -> (w384:refnum<vi>)
        n252 = control-ref of="自定义 2"() -> (w381:refnum<vi>)
        n253 = control-ref of="自定义"() -> (w382:refnum<vi>)
        n254 = Build Array(w379, w378) -> (w377:refnum<vi>[])
        n255 = Build Array(w384, w380, w381, w382) -> (w383:refnum<vi>[])
        n256 = for {
          tunnel: w377 -> [w385] mode=indexing
          n257 = invoke class="下拉列表 (严格)" method="Reinit To Default"(reference=w385) -> ()  [unwired: 2 in, 3 out]
        }
        n258 = for {
          tunnel: w383 -> [w386] mode=indexing
          n259 = invoke class="Clust" method="Reinit To Default"(reference=w386) -> ()  [unwired: 2 in, 3 out]
        }
      }
      event "确定": Value Change {
        w387 = TRUE
        n260 = event-data() -> ()  [unwired: 1 in, 6 out]
      }
      event "退出": Value Change; Panel Close {
        n261 = event-data() -> ()  [unwired: 1 in, 3 out]
      }
    }
  }
  "确定输出" <- w14
